vi "RT_Control_Adrian_MicrophonesWithAngle.vi"(10 "rt fifo":refnum<k33>, 11 "Parameters":T1={"N_chan"=0, "Input Rate (Hz)"=0.0, "Acq Time (s)"=0.0, "NumOfWarmupIters"=0, "Size fifo"=0, "Period NCL (ms)"=0, "Timeout fifo Read"=0, "Size Sent Array"=0, "Output offsets"=[], "Input offsets"=[0.0, 0.0, 0.0, 0.0, 0.0, 0.0, 0.0, 0.0]}) -> (0 "error out":errorcluster, 2 "Delayed Cycles":dbl)   [LabVIEW 2021]
uses:
  parametersRT.ctl
  <vilib>/DAQmx/write.llb/DAQmx Write (Analog 1D DBL NChan 1Samp).vi
  <vilib>/DAQmx/read.llb/DAQmx Read (Analog 1D DBL NChan 1Samp).vi
  <vilib>/DAQmx/read.llb/DAQmx Read (Digital 2D U32 NChan NSamp).vi
  <vilib>/Analysis/baseanly.llb/Mean (DBL).vi
  <vilib>/DAQmx/configure/timing.llb/DAQmx Timing (Sample Clock).vi
  <vilib>/DAQmx/miscellaneous.llb/DAQmx Fill In Error Info.vi
  <resource>/objmgr/daqmx.rc
  <vilib>/Analysis/NI_AALBase.lvlib
panel:
  out "Encoder Raw Outputs":dbl[][](array[numeric])
  out "Encoder Mean Outputs":dbl[](array[numeric])
  in  "F_Loop":dbl=100.0
  in  "Fs_DC":dbl=5000.0
  in  "Zero Angle":dbl[](array[numeric])=[-16.79, 2.64, -15.0, 3.7]
  out "data":dbl[](array[numeric]) format="%0.2f"
  out "Numeric":i32
  out "output array":dbl[](array[numeric])
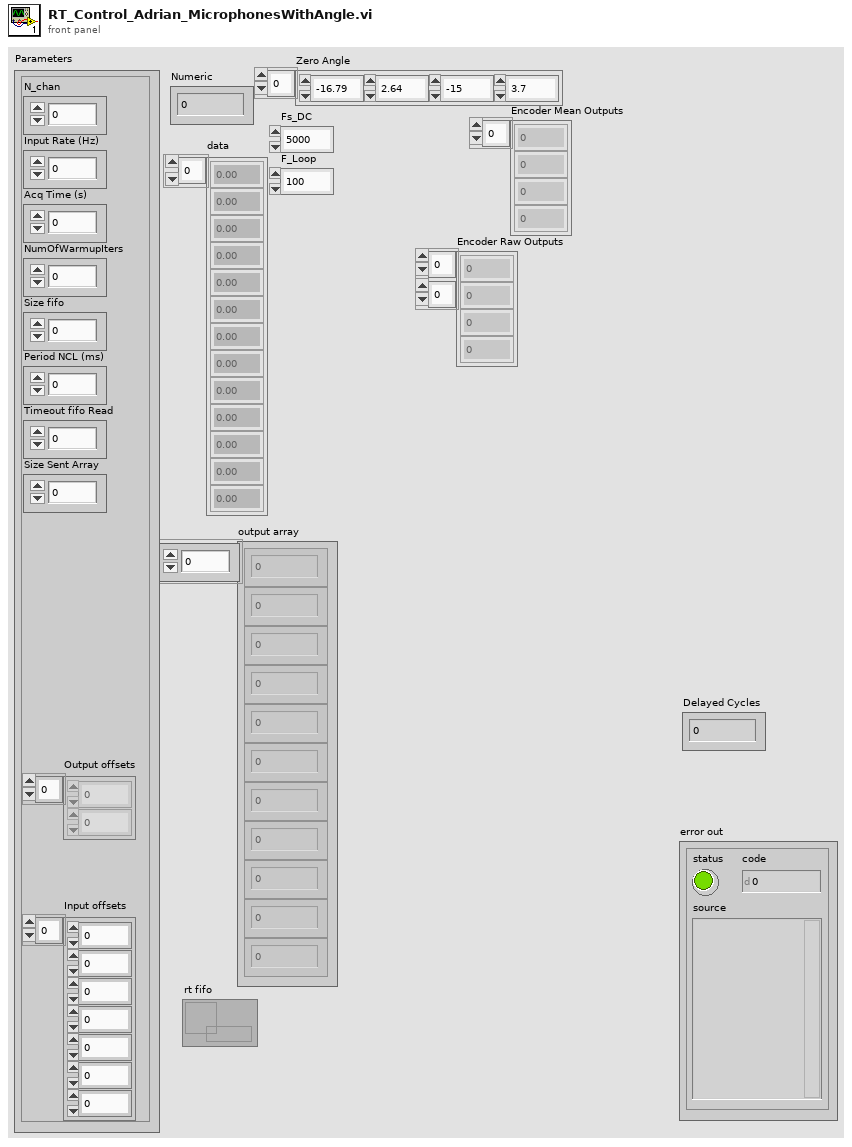
[diagram p1: front panel]
types:
  T1 = typedef "parametersRT.ctl" = cluster{"N_chan":u32, "Input Rate (Hz)":dbl, "Acq Time (s)":dbl, "NumOfWarmupIters":u32, "Size fifo":u32, "Period NCL (ms)":i64, "Timeout fifo Read":i32, "Size Sent Array":i32, "Output offsets":dbl[], "Input offsets":dbl[]}
  T2 = cluster{"Csn task out":refnum<k21>, "CLK task out":refnum<k21>, "D0 task out":refnum<k21>}
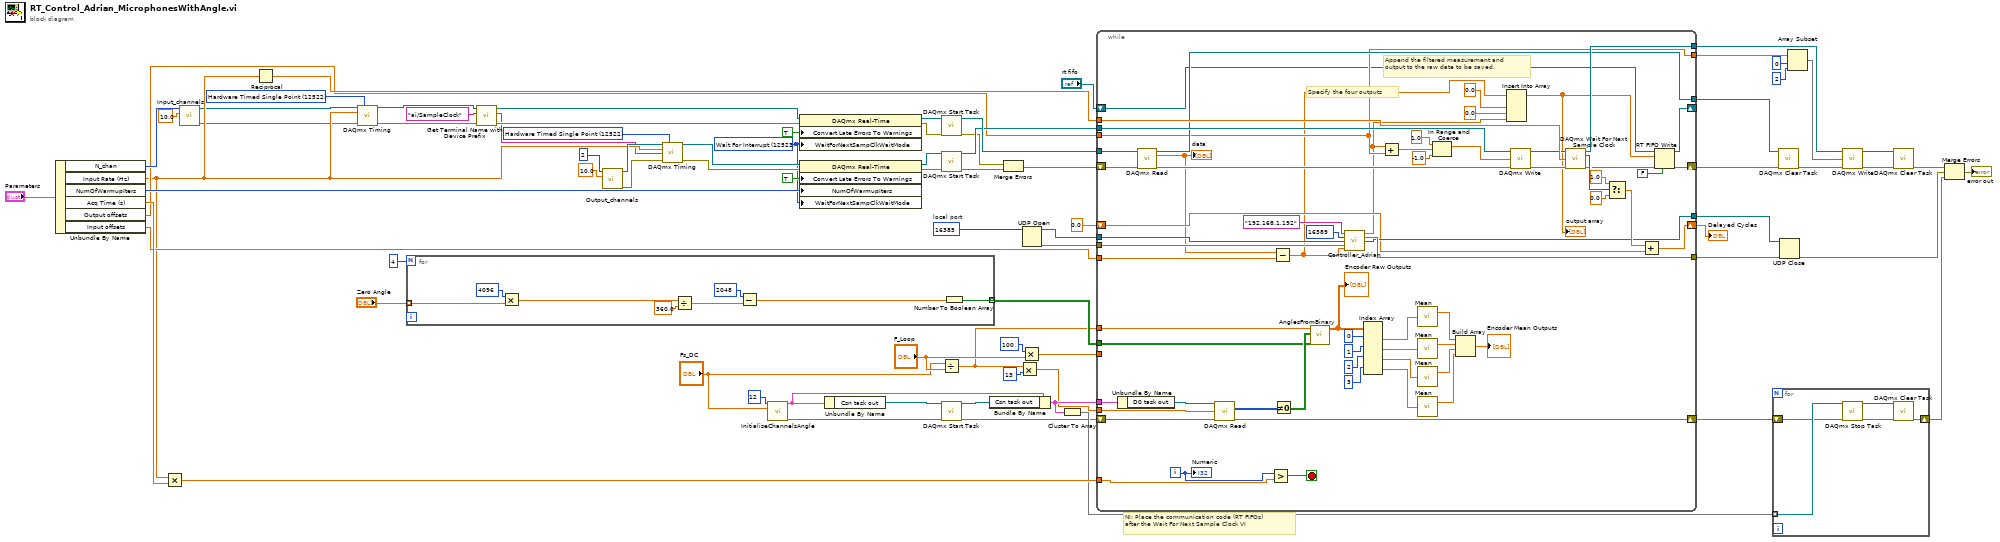
[diagram p0: block diagram]
diagram:
  w36 = u16 16385  # local port
  w43 = 12522 items=["Finite Samples"=10178, "Continuous Samples"=10123, "Hardware Timed Single Point"=12522] ("sample mode")
  w52 = 12523 items=["Wait For Interrupt"=12523, "Poll"=12524, "Yield"=12525] ("WaitForNextSampClkWaitMode")
  w78 = 12522 items=["Finite Samples"=10178, "Continuous Samples"=10123, "Hardware Timed Single Point"=12522] ("sample mode")
  # "NI: Place the communication code (RT FIFOs) \nafter the Wait For Next Sample Clock VI"
  n1 = Unbundle By Name("Parameters") -> ("N_chan"=w63:u32, "Input Rate (Hz)"=w47:dbl, "NumOfWarmupIters"=w64:u32, "Acq Time (s)"=w71:dbl, "Output offsets"=w62:dbl[], "Input offsets"=w53:dbl[])
  n2 = Multiply(x=w47, y=w71) -> (x*y=w30:dbl)
  n3 = call "Input_channels.vi"("Range"=10.0, "nchan"=w63) -> ("error out"=w45:errorcluster, "Refnum out"=w44:refnum<k21>)  [unwired: 8 in]
  n4 = Reciprocal(x=w47) -> (1/x=w77:dbl)
  n5 = call-poly <vilib>:"DAQmx Timing.vi"("task/channels in"=w44, "sample mode"=w43, "rate"=w47, "error in"=w45) -> ("task out"=w24:refnum<k21>, "error out"=w26:errorcluster)  [unwired: 10 in]
  n6 = for {
    N: 4 -> [_]
    tunnel: [w83] -> w5 mode=indexing
    tunnel: "Zero Angle" -> [w86] mode=indexing
    n7 = Multiply(x=4096, y=w86) -> (x*y=w87:dbl)
    n8 = Divide(x=w87, y=360.0) -> (x/y=w81:dbl)
    n9 = Subtract(x=2048, y=w81) -> (x-y=w80:dbl)
    n10 = Number To Boolean Array(number=w80) -> (Boolean array=w83:bool[])
  }
  n11 = call "Get Terminal Name with Device Prefix.vi"("error in (no error)"=w26, "Local Terminal Name"="ai/SampleClock", "task/channels in"=w24) -> ("error out"=w25:errorcluster, "Terminal Name with Device Prefix"=w22:tag, "task out"=w23:refnum<k21>)  [unwired: 6 in]
  n12 = call "Output_channels.vi"("Range"=10.0 ("Maximum Value"), "nchan"=2) -> ("error out"=w68:errorcluster, "Refnum out"=w67:refnum<k21>)  [unwired: 8 in]
  n13 = call-poly <vilib>:"DAQmx Timing.vi"("task/channels in"=w67, "sample mode"=w78, "rate"=w47, "source"=w22, "error in"=w68) -> ("task out"=w76:refnum<k21>, "error out"=w75:errorcluster)  [unwired: 9 in]
  n14 = call "InitialiseChannelsAngle.vi"("Number of data bits"=12, "Fs"="Fs_DC") -> ("output cluster"=w10:T2, "error out"=w11:errorcluster)  [unwired: 12 in]
  n15 = property class="DAQmx Real-Time"(reference=w23, error in=w25, "Convert Late Errors To Warnings"=TRUE, "WaitForNextSampClkWaitMode"=w52) -> (reference out=w40:refnum<k21>, error out=w39:errorcluster)
  n16 = property class="DAQmx Real-Time"(reference=w76, error in=w75, "Convert Late Errors To Warnings"=TRUE, "NumOfWarmupIters"=w64, "WaitForNextSampClkWaitMode"=w52) -> (reference out=w72:refnum<k21>, error out=w49:errorcluster)
  n17 = Unbundle By Name(w10) -> ("Csn task out"=w18:refnum<k21>)
  n18 = call <vilib>:"DAQmx Start Task.vi"("task/channels in"=w40, "error in"=w39) -> ("task out"=w70:refnum<k21>, "error out"=w38:errorcluster)  [unwired: 12 in]
  n19 = call <vilib>:"DAQmx Start Task.vi"("task/channels in"=w72, "error in"=w49) -> ("task out"=w69:refnum<k21>, "error out"=w48:errorcluster)  [unwired: 12 in]
  n20 = Divide(x="Fs_DC", y="F_Loop") -> (x/y=w3:dbl)
  n21 = call <vilib>:"DAQmx Start Task.vi"("task/channels in"=w18, "error in"=w11) -> ("task out"=w17:refnum<k21>, "error out"=w6:errorcluster)  [unwired: 12 in]
  n22 = Bundle By Name(cluster=w10, "Csn task out"=w17) -> (w2:T2)
  n23 = Merge Errors(w38, w48) -> (w37:errorcluster)
  n24 = Multiply(x=w3, y=13) -> (x*y=w1:dbl)
  n25 = Multiply(x=100, y="F_Loop") -> (x*y=w4:dbl)
  n26 = UDP Open(11:w36) -> (port=w34:refnum<k16>, 0:w35:errorcluster)  [unwired: 4 in, 1 out]
  n27 = Cluster To Array(cluster=w2) -> (array=w9:refnum<k21>[])
  n28 = while {
    shift-right: [w118] -> w46
    shift-left: w37 -> [w136]
    shift-right: [w148] -> w79
    shift-left: 0.0 ("f") -> [w123]
    tunnel: w77 -> [w146]
    tunnel: w30 -> [w144]
    tunnel: w69 -> [w142]
    tunnel: [w137] -> w73
    tunnel: w70 -> [w138]
    tunnel: [w140] -> w61
    tunnel: w62 -> [w131]
    tunnel: [w131] -> w56
    tunnel: w53 -> [w139]
    tunnel: w35 -> [w129]
    tunnel: w34 -> [w128]
    tunnel: [w127] -> w33
    tunnel: [w126] -> w32
    shift-right: [w114] -> _
    shift-left: "rt fifo" -> [w115]
    shift-right: [w93] -> w7
    shift-left: w6 -> [w92]
    tunnel: w5 -> [w91]
    tunnel: w4 -> [_]
    tunnel: w3 -> [w90]
    tunnel: w2 -> [w89]
    tunnel: w1 -> [w88]
    i -> [w121]
    stop <- w145 stop-if-true
    # "Append the filtered measurement and \noutput to the raw date to be saved."
    # "Specify the four outputs"
    n29 = Unbundle By Name(w89) -> ("D0 task out"=w110:refnum<k21>)
    n30 = call-poly <vilib>:"DAQmx Read.vi"("task/channels in"=w138, "error in"=w136) -> ("task out"=w137:refnum<k21>, "data"=w120:dbl[], "error out"=w135:errorcluster)  [unwired: 11 in]
    "data" <- w120
    n31 = call-poly <vilib>:"DAQmx Read.vi"("task/channels in"=w110, "number of samples per channel"=w88, "error in"=w92) -> ("data"=w109:u32[][], "error out"=w93:errorcluster)  [unwired: 10 in, 1 out]
    n32 = Greater?(x=w121, y=w144) -> (0:w145:bool)
    n33 = Subtract(x=w120, y=w139) -> (x-y=w122:dbl[])
    n34 = Not Equal To 0?(x=w109) -> (x != 0?=w108:bool[][])
    n35 = call "AnglesFromBinary.vi"("Binary Offset"=w91, "Array"=w108, "Buffer Length"=w90) -> ("Unwrapped Phase"=w107:dbl[][])  [unwired: 8 in]
    "Encoder Raw Outputs" <- w107
    n36 = call "Controller_Adrian.vi"("name 2"="192.168.1.192", "port or service name"=u16 16389, "connection ID"=w128, "error in (no error)"=w129, "x"=w122) -> ("*(type *) &x"=w113:dbl[], "error out"=w127:errorcluster, "connection ID out"=w126:refnum<k16>)  [unwired: 8 in]
    n37 = Index Array(array=w107, index (row) #1=0 ("index (row)"), index (row) #2=1 ("index (row)"), index (row) #3=2 ("index (row)"), index (row) #4=3 ("index (row)")) -> (element #1=w102:dbl[], element #2=w101:dbl[], element #3=w100:dbl[], element #4=w99:dbl[])  [unwired: 4 in]
    n38 = Add(x=w113, y=w131) -> (x+y=w133:dbl[])
    n39 = call-poly <vilib>:"Mean.vi"("X"=w102) -> ("mean"=w95:dbl)  [unwired: 1 out]
    n40 = call-poly <vilib>:"Mean.vi"("X"=w101) -> ("mean"=w96:dbl)  [unwired: 1 out]
    n41 = call-poly <vilib>:"Mean.vi"("X"=w100) -> ("mean"=w97:dbl)  [unwired: 1 out]
    n42 = call-poly <vilib>:"Mean.vi"("X"=w99) -> ("mean"=w98:dbl)  [unwired: 1 out]
    n43 = In Range and Coerce(upper limit=1.0, x=w133, lower limit=-1.0) -> (coerced(x)=w130:dbl[])  [unwired: 1 out]
    n44 = Build Array(w95, w96, w97, w98) -> (→"Encoder Mean Outputs":dbl[])
    n45 = Insert Into Array(array=w122, new element #1=0.0 ("new element/subarray"), new element #2=0.0 ("new element/subarray"), new element #3=w113) -> (w116:dbl[])  [unwired: 1 in]
    "output array" <- w116
    n46 = call-poly <vilib>:"DAQmx Write.vi"("task/channels in"=w142, "data"=w130, "error in"=w135) -> ("task out"=w141:refnum<k21>, "error out"=w143:errorcluster)  [unwired: 10 in, 1 out]
    n47 = call <vilib>:"DAQmx Wait For Next Sample Clock.vi"("task/channels in"=w141, "timeout (sec)"=w146, "error in"=w143) -> ("task out"=w140:refnum<k21>, "is late?"=w147:bool, "error out"=w117:errorcluster)  [unwired: 10 in]
    n48 = Select(t=1.0, s=w147, f=0.0) -> (s? t:f=w149:dbl)
    n49 = Add(x=w149, y=w123) -> (x+y=w148:dbl)
    n50 = RT FIFO Write(0:w115, 1:w116, 3:w117, 5:FALSE ("overwrite on timeout (T)")) -> (8:w114:refnum<k33>, 11:w118:errorcluster)  [unwired: 1 in, 2 out]
    "Numeric" <- w121
  }
  "Delayed Cycles" <- w79
  n51 = for {
    tunnel: w9 -> [w156] mode=indexing
    shift-right: [w152] -> w8
    shift-left: w7 -> [w154]
    n52 = call <vilib>:"DAQmx Stop Task.vi"("task/channels in"=w156, "error in"=w154) -> ("task out"=w155:refnum<k21>, "error out"=w153:errorcluster)  [unwired: 12 in]
    n53 = call <vilib>:"DAQmx Clear Task.vi"("task in"=w155, "error in"=w153) -> ("error out"=w152:errorcluster)  [unwired: 13 in]
  }
  n54 = call <vilib>:"DAQmx Clear Task.vi"("task in"=w73, "error in"=w46) -> ("error out"=w59:errorcluster)  [unwired: 13 in]
  n55 = UDP Close(connection ID=w32, 8:w33) -> (error out=w31:errorcluster)  [unwired: 1 out]
  n56 = Array Subset(array=w56, index=0, length=2) -> (w57:dbl[])
  n57 = call-poly <vilib>:"DAQmx Write.vi"("task/channels in"=w61, "data"=w57, "error in"=w59) -> ("task out"=w60:refnum<k21>, "error out"=w58:errorcluster)  [unwired: 10 in, 1 out]
  n58 = call <vilib>:"DAQmx Clear Task.vi"("task in"=w60, "error in"=w58) -> ("error out"=w51:errorcluster)  [unwired: 13 in]
  n59 = Merge Errors(w51, w31, w8) -> (→"error out":errorcluster)
